vi "Microwave Freq Scan.vi"(8 "error in (no error)":errorcluster, 10 "Microwave.lvclass":refnum<class "Microwave.lvclass">, 11 "Microwave Freq Scan in":refnum<class "Microwave Freq Scan.lvclass">) -> (0 "error out":errorcluster, 3 "Microwave Freq Scan out":refnum<class "Microwave Freq Scan.lvclass">)   [LabVIEW 2015, in "Microwave Freq Scan.lvclass"]
uses:
  Microwave Freq Scan.lvclass
  Instruments/Microwave/Microwave.lvclass
  Scanner/Scanner.lvclass
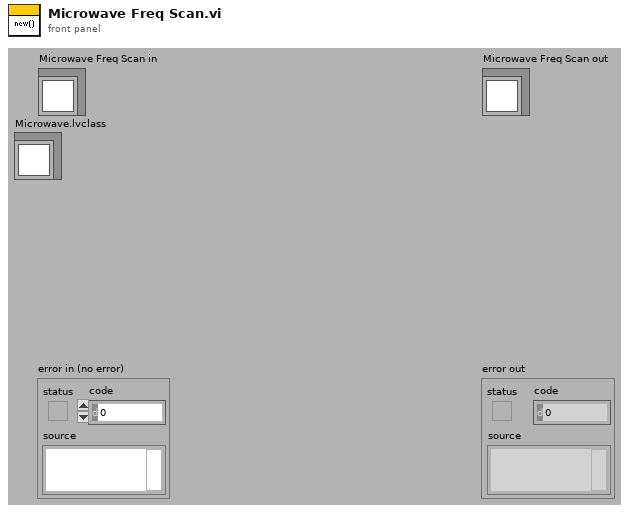
[diagram p1: front panel]
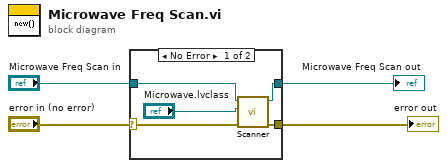
[diagram p0: block diagram]
diagram:
  n1 = case shown="No Error" "error in (no error)" {
    selector: "error in (no error)" -> [w6 w11]
    tunnel: [w5 w11] -> w3
    tunnel: [w8 w10] -> w1
    tunnel: "Microwave Freq Scan in" -> [w9 w10]
    frame No Error {
      n2 = call "Scanner.vi"("error in (no error)"=w6, "Scannable"="Microwave.lvclass", "Scanner.lvclass in"=w9) -> ("error out"=w5:errorcluster, "Scanner.lvclass out"=w8:refnum<class "Microwave Freq Scan.lvclass">)  [unwired: 1 in, 6 out]
    }
    frame Error {
    }
  }
  "error out" <- w3
  "Microwave Freq Scan out" <- w1
